vi "test_fpga_scanEngineCore.vi"() -> ()   [LabVIEW 2016]
uses:
  <vilib>/Platform/TimedLoop/XDataNode/wakeup.ctl
  <vilib>/Platform/TimedLoop/XDataNode/XDNodeRunTimeDep.lvlib
  <vilib>/Platform/TimedLoop/XDataNode/nitl_modes.ctl
  <vilib>/Platform/TimedLoop/XDataNode/timing_clust.ctl
  <vilib>/Platform/TimedLoop/XDataNode/XDataNode.xnode
  <vilib>/eio/EIONode/EIONode.xnode
  <vilib>/rvi/FXPMathLib/FxpInterpret/XNode/nifxpmath_Interpret.xnode
  <instrlib>/_niInstr/Basic Elements/v1/FPGA/niInstr Basic Elements v1 FPGA.lvlib
  <vilib>/rvi/FXPMathLib/FxpSub/XNode/nifxpmath_Sub.xnode
  <vilib>/rvi/FXPMathLib/sim/FxpSim.dll
  <vilib>/rvi/FXPMathLib/FxpMul/XNode/nifxpmath_Multiplier.xnode
  <vilib>/rvi/FXPMathLib/FxpAdd/XNode/nifxpmath_Add.xnode
  <vilib>/rvi/DataTransferAndStorage/Container/XNode/niFpgaContainer.xnode
  <vilib>/rvi/FIFO/Fifo_Resource/nirvififoEmulationWrite.vi
  <vilib>/rvi/eio/common/nirviEmuTemplateMethod_errors.vi
  <vilib>/rvi/DataTransferAndStorage/Register/Emulation/niFpgaRegisterEmulation.vi
panel:
  out "pixelEvent":bool
  out "fastIndices":cluster{"index":u16, "next":u16}
  out "indices":T1
  out "outputValid":cluster{"scanValid":bool, "slowValid":bool}
  in  "doSlowMoveFIFO":bool
  out "output":T2
  out "clocks":T3
  out "savedPoint":T4
  out "slowIndices":cluster{"index":u16, "f":u16}
  in  "scanEnabled":bool
  in  "fastDecFactorInv":fxp<+,16,0>
  in  "slowUpStep":fxp<+,22,0>
  in  "outWaveSizeSlow":u16
  in  "scanOffset":cluster{"x":fxp<+/-,16,1>, "y":fxp<+/-,16,1>}
  in  "singleDirectionScan":bool
  in  "moveToPoint":cluster{"x":fxp<+/-,16,1>, "y":fxp<+/-,16,1>}
  in  "invMoveToDec":fxp<+,16,0>
  out "slowMoving":bool
  in  "outputMatrix":T5
  in  "frioRecordingEnable":bool=TRUE
  in  "scanSize":T6
  in  "scanRates":T7={"outputRate"=50, "fastDecFactor"=0, "outWaveSizeFast"=0, "pplUpsampling"=0, "numLines"=0}
  in  "moveRates":T8
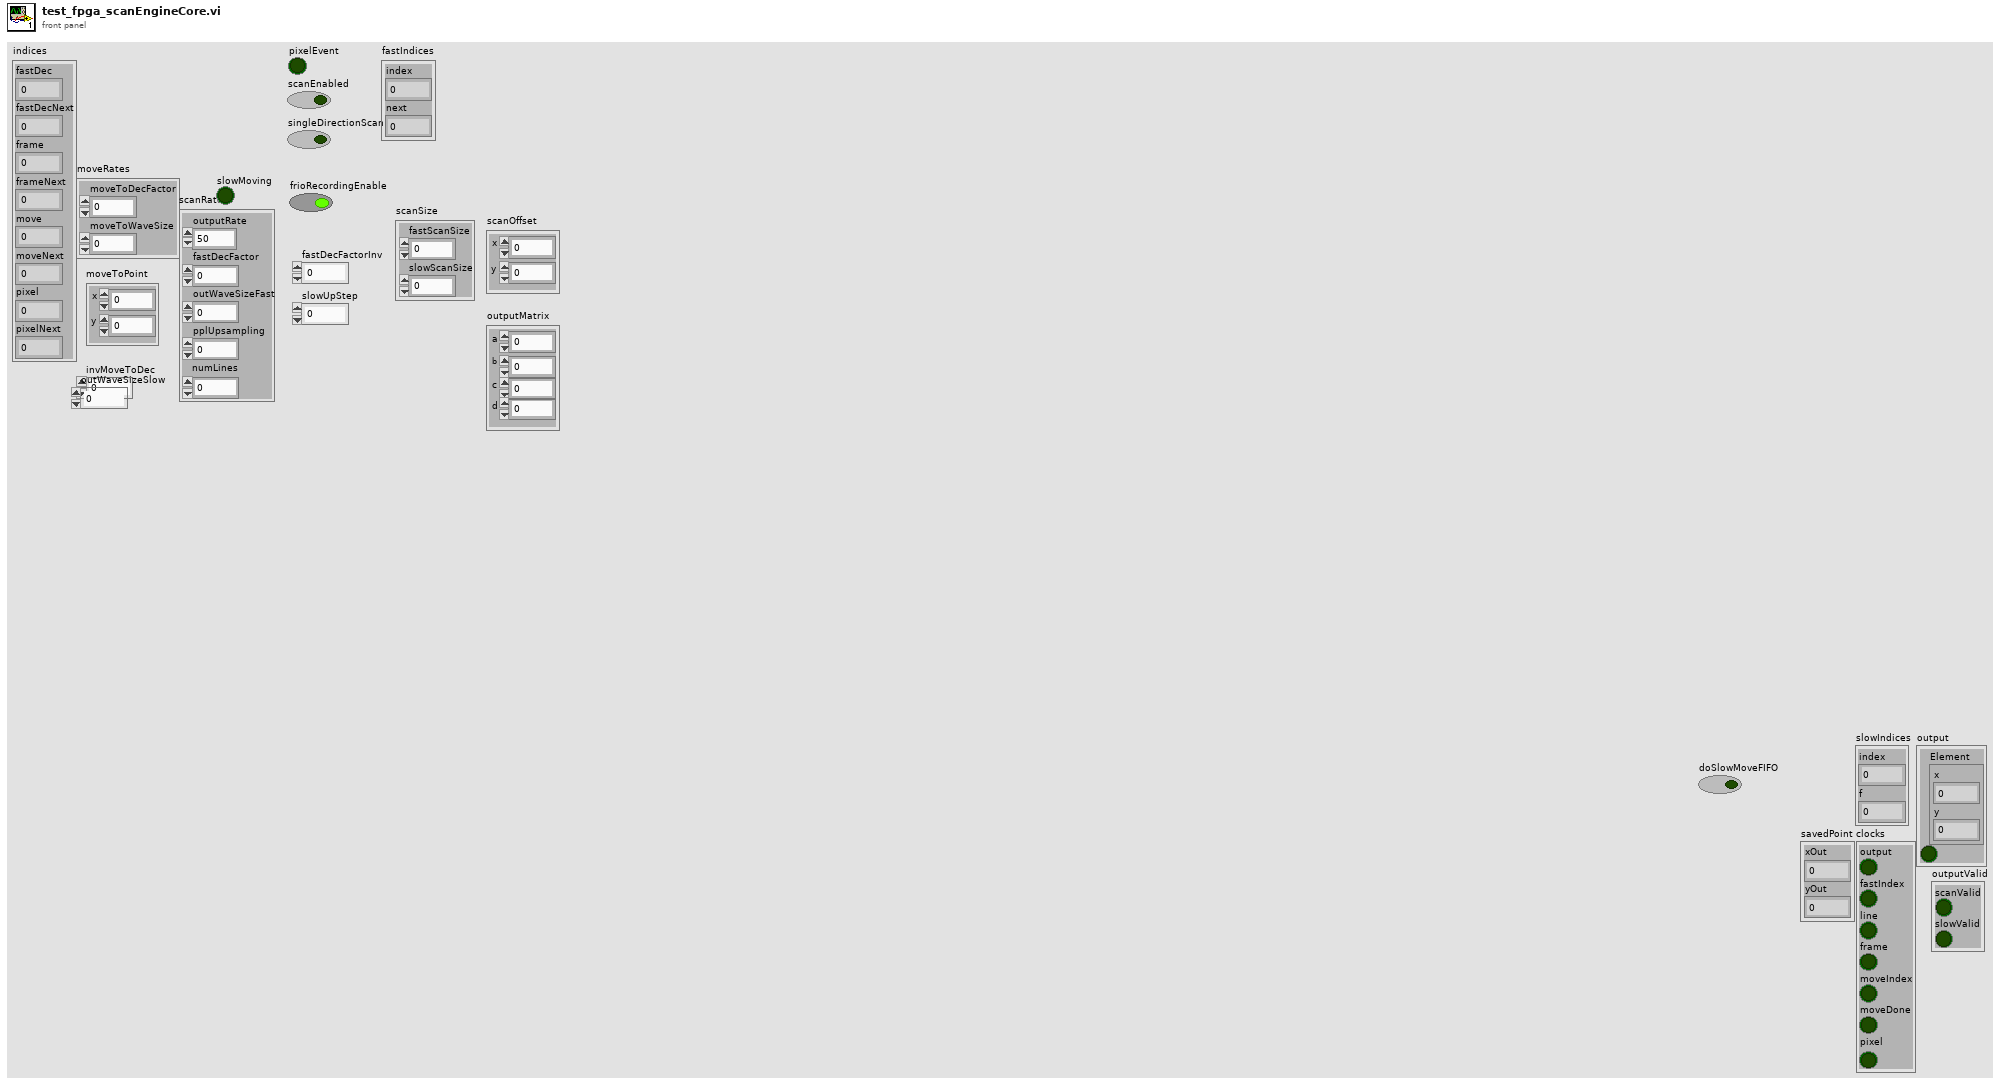
[diagram p1: front panel]
types:
  T1 = cluster{"fastDec":u16, "fastDecNext":u16, "frame":u16, "frameNext":u16, "move":u16, "moveNext":u16, "pixel":u16, "pixelNext":u16}
  T2 = cluster{"Element":cluster{"x":i16, "y":i16}, bool}
  T3 = cluster{"output":bool, "fastIndex":bool, "line":bool, "frame":bool, "moveIndex":bool, "moveDone":bool, "pixel":bool}
  T4 = cluster{"xOut":fxp<+/-,18,2>, "yOut":fxp<+/-,18,2>}
  T5 = cluster{"a":fxp<+/-,18,2>, "b":fxp<+/-,18,2>, "c":fxp<+/-,18,2>, "d":fxp<+/-,18,2>}
  T6 = cluster{"fastScanSize":fxp<+,17,1>, "slowScanSize":fxp<+,17,1>}
  T7 = cluster{"outputRate":u16, "fastDecFactor":u16, "outWaveSizeFast":u16, "pplUpsampling":u16, "numLines":u16}
  T8 = cluster{"moveToDecFactor":u16, "moveToWaveSize":u16}
  T9 = typedef "XDNodeRunTimeDep.lvlib/timing_clust.ctl" = cluster{"Expected End [f-1]":u64, "Actual End [f-1]":u64, "Finished Late? [f-1]":bool, "Expected End [i-1]":u64, "Actual End [i-1]":u64, "Finished Late? [i-1]":bool, "Expected Start [i]":u64, "Actual Start [i]":u64, "Expected Start [f]":u64, "Actual Start [f]":u64, "Source Name":string, "Structure Name":string, "Period":i64, "Deadline":i64, "Offset":i64, "Start":i64, "Priority":i32, "Timeout":i32, "Mode":T10, "Wakeup Reason":T11, "Error":errorcluster, "Source Type":string, "Secondary Source Type":string, "Global End Time":u64, "Global Start Time":u64, "Frame Duration":u64, "Iteration Duration":u64, "Assigned CPU":i32, "I/O Scan Engine Mode":u32}
  T10 = typedef "XDNodeRunTimeDep.lvlib/nitl_modes.ctl" = enum32{"No Change", "Process missed periods, maintain original phase", "Discard missed periods, maintain original phase", "Process missed periods, ignore original phase", "Discard missed periods, ignore original phase"}
  T11 = typedef "XDNodeRunTimeDep.lvlib/wakeup.ctl" = enum32{"Normal", "Aborted", "Asynchronous wakeup", "Timing source error", "Timed loop error", "Timeout"}
  T12 = cluster{"fastDec":u16, "fastDecNext":u16, "frame":u16, "frameNext":u16, "move":u16, "moveNext":u16, "pixel":u16, "pixelNext":u16, "blanking":u32, "blankingNext":u32}
  T13 = cluster{"index":u16, "next":u16, "blanking":u32, "blankingNext":u32}
  T14 = cluster{"x-y":fxp<+/-,18,2>, "x-y":fxp<+/-,18,2>}
  T15 = cluster{"interpOutput":fxp<+/-,19,2>, "interpOutput":fxp<+/-,19,2>}
  T16 = cluster{"x+y":fxp<+/-,18,2>, "x+y":fxp<+/-,18,2>}
  T17 = cluster{"edge detected":bool, "output valid":bool}
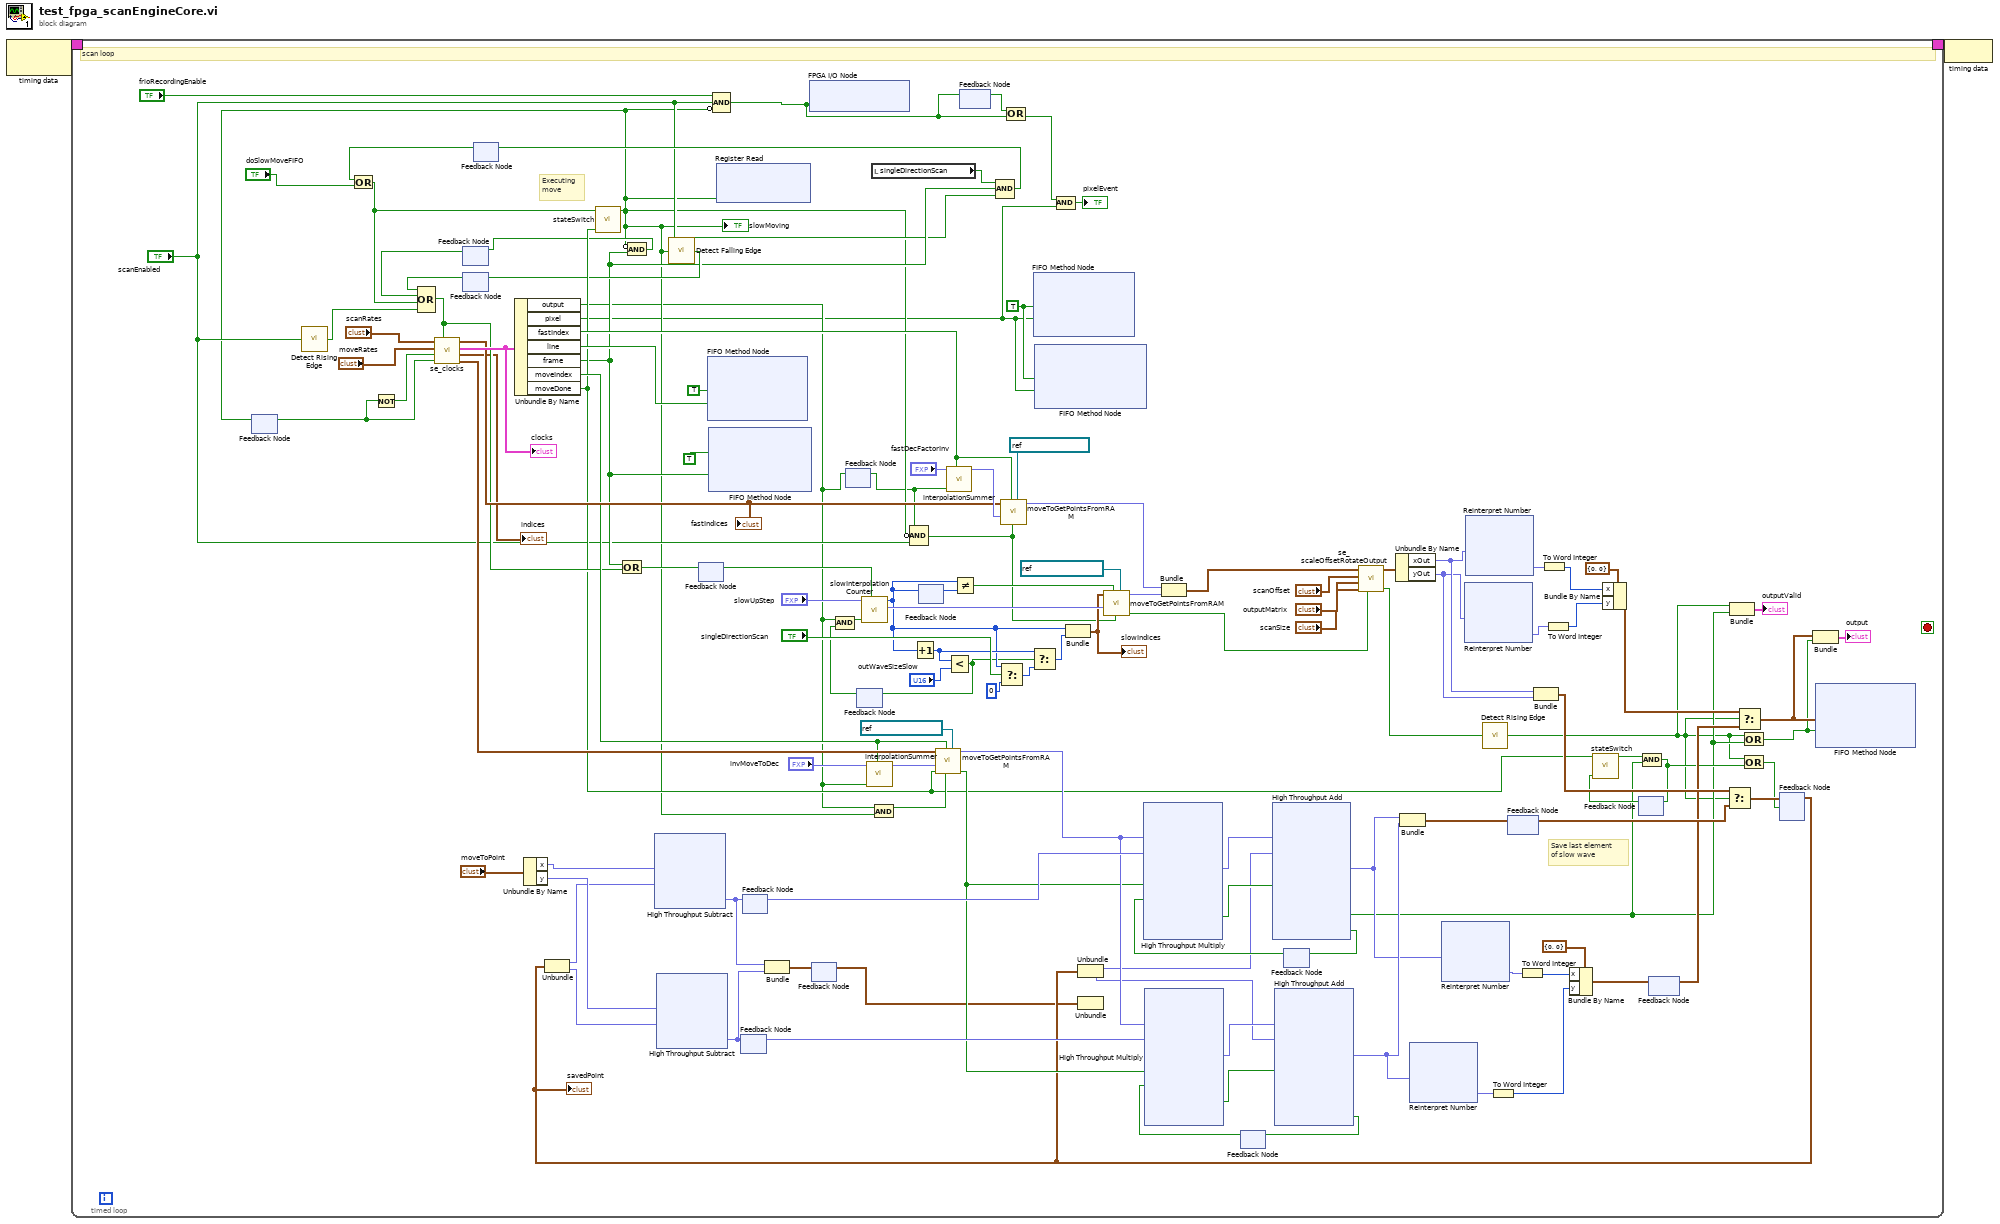
[diagram p0: block diagram]
diagram:
  n1 = node-c288() -> (w2:T9)  [unwired: 1 in]
  n2 = timed-loop {
    timing: w2 -> [_]
    timing-out: [_] -> w1
    stop <- _ stop-if-true
    w82 = TRUE ("Element")
    # "Save last element \nof slow wave"
    # "Executing\nmove"
    # "scan loop"
    n3 = feedback #1() -> (w17:bool)  [unwired: 1 in]
    n4 = call <instrlib>:"Detect Rising Edge.vi"("signal"="scanEnabled") -> ("edge detected"=w65:bool)  [unwired: 14 in]
    n5 = Not(x=w17) -> (.not. x?=w16:bool)
    n6 = feedback #2() -> (w64:bool)  [unwired: 1 in]
    n7 = feedback #3() -> (w63:bool)  [unwired: 1 in]
    n8 = feedback #4() -> (w33:bool)  [unwired: 1 in]
    n9 = Compound Arithmetic op=OR(w33, "doSlowMoveFIFO") -> (w28:bool)
    n10 = Compound Arithmetic op=OR(w63, w64, w28, w65) -> (w31:bool)
    n11 = call "se_clocks.vi"("se.p.resetClocks"=w31, "stepSlow"=w17, "stepScan"=w16, "moveRates"="moveRates", "se.p.clocks"="scanRates") -> ("moveIndices"=w73:cluster{"index":u16, "next":u16}, "indices"=→"indices":T12, "clocks"=w77:T3, "fastIndices"=w75:T13)  [unwired: 3 in]
    "clocks" <- w77
    "fastIndices" <- w75
    n12 = Unbundle By Name(w77) -> ("output"=w9:bool, "pixel"=w7:bool, "fastIndex"=w72:bool, "line"=w76:bool, "frame"=w27:bool, "moveIndex"=w71:bool, "moveDone"=w30:bool)
    n13 = Unbundle By Name("moveToPoint") -> ("x"=w103:fxp<+/-,16,1>, "y"=w104:fxp<+/-,16,1>)
    n14 = call "stateSwitch.vi"("disable"=w30, "enable"=w28) -> ("state"=w14:bool)  [unwired: 9 in]
    "slowMoving" <- w14
    n15 = feedback-in #1(w14) -> ()
    n16 = Compound Arithmetic op=OR(w27, w31) -> (w32:bool)
    n17 = Compound Arithmetic op=AND(invert w14, w27) -> (w26:bool)
    n18 = feedback-in #2(w26) -> ()
    n19 = call <instrlib>:"Detect Falling Edge.vi"("signal"=w14) -> ("edge detected"=w29:bool)  [unwired: 14 in]
    n20 = feedback-in #3(w29) -> ()
    n21 = feedback-in #5(w32) -> ()
    n22 = feedback #5() -> (w10:bool)  [unwired: 1 in]
    n23 = xnode ("FIFO Method Node")("Element"=TRUE, "Input Valid"=w76) -> ()  [unwired: 1 in, 2 out]
    n24 = xnode ("FIFO Method Node")("Element"=TRUE, "Input Valid"=w27) -> ()  [unwired: 1 in, 2 out]
    n25 = Compound Arithmetic op=AND("frioRecordingEnable", "scanEnabled", invert w14) -> (w4:bool)
    n26 = xnode ("Register Read")("Data"=w14) -> ()  [unwired: 1 in, 1 out]
    n27 = feedback #6() -> (w114:fxp<+/-,18,2>)  [unwired: 1 in]
    n28 = feedback #7() -> (w111:fxp<+/-,18,2>)  [unwired: 1 in]
    n29 = xnode "FPGA I/O Node"("outputEnabled"=w4) -> ()  [unwired: 1 in, 1 out]
    n30 = feedback #8() -> (w43:T14)  [unwired: 1 in]
    n31 = feedback #9() -> (w8:bool)  [unwired: 1 in]
    n32 = feedback-in #9(w9) -> ()
    n33 = feedback #10() -> (w11:bool)  [unwired: 1 in]
    n34 = Compound Arithmetic op=AND(w9, w11) -> (w13:bool)
    n35 = call "slowInterpolationCounter.vi"("reset"=w10, "doStep"=w13, "upStep"="slowUpStep") -> ("fraction"=w80:fxp<+,28,0>, "index"=w67:u16)  [unwired: 7 in]
    n36 = call "interpolationSummer.vi"("reset"=w71, "doStep"=w9, "upStep"="invMoveToDec") -> ("position"=w98:fxp<+,22,0>)  [unwired: 8 in]
    n37 = local read "singleDirectionScan"() -> (w35:bool)
    n38 = Compound Arithmetic op=AND(w9, w14) -> (w42:bool)
    n39 = Compound Arithmetic op=AND(w8, invert w14, "scanEnabled") -> (w41:bool)
    n40 = Increment(x=w67) -> (x+1=w95:u16)
    n41 = feedback-in #11(w67) -> ()
    n42 = feedback #11() -> (w68:u16)  [unwired: 1 in]
    n43 = call "moveToGetPointsFromRAM.vi"("Memory In"=refnum<k21> "moveToWave", "inputValid"=w42, "reset"=w71, "maxReached"=w30, "interpPosition"=w98, "adresses"=w73) -> ("outputValid"=w51:bool, "interpOutput"=w97:fxp<+/-,19,2>)  [unwired: 4 in]
    n44 = call "interpolationSummer.vi"("reset"=w72, "doStep"=w8, "upStep"="fastDecFactorInv") -> ("position"=w87:fxp<+,22,0>)  [unwired: 8 in]
    n45 = Less?(x=w95, y="outWaveSizeSlow") -> (x < y?=w12:bool)
    n46 = feedback-in #10(w12) -> ()
    n47 = Not Equal?(x=w67, y=w68) -> (x != y?=w66:bool)
    n48 = feedback-in #12(w4) -> ()
    n49 = feedback #12() -> (w3:bool)  [unwired: 1 in]
    n50 = Compound Arithmetic op=AND(w35, w27, "scanEnabled") -> (w34:bool)
    n51 = feedback-in #4(w34) -> ()
    n52 = Select(t=w67, s="singleDirectionScan", f=u16 0) -> (s? t:f=w94:u16)
    n53 = call "moveToGetPointsFromRAM.vi"("Memory In"=refnum<k21> "fastAxisWave", "inputValid"=w41, "reset"=w72, "interpPosition"=w87, "adresses"=w75) -> ("interpOutput"=w85:fxp<+/-,19,2>)  [unwired: 5 in, 1 out]
    n54 = Compound Arithmetic op=OR(w3, w4) -> (w5:bool)
    n55 = Select(t=w95, s=w12, f=w94) -> (s? t:f=w81:u16)
    n56 = xnode ("FIFO Method Node")("Element"=w82, "Input Valid"=w7) -> ()  [unwired: 1 in, 2 out]
    n57 = xnode ("FIFO Method Node")("Element"=w82, "Input Valid"=w7) -> ()  [unwired: 1 in, 2 out]
    n58 = Compound Arithmetic op=AND(w5, w7) -> (→"pixelEvent":bool)
    n59 = Bundle("index"=w67, "f"=w81) -> (w69:cluster{"index":u16, "f":u16})  [unwired: 1 in]
    "slowIndices" <- w69
    n60 = Unbundle(w43) -> ()  [unwired: 2 out]
    n61 = call "moveToGetPointsFromRAM.vi"("Memory In"=refnum<k21> "slowAxisWave", "inputValid"=w41, "reset"=w66, "interpPosition"=w80, "adresses"=w69) -> ("outputValid"=w70:bool, "interpOutput"=w84:fxp<+/-,19,2>)  [unwired: 5 in]
    n62 = Bundle("interpOutput"=w85, "interpOutput"=w84) -> (w83:T15)  [unwired: 1 in]
    n63 = feedback #13() -> (w107:bool)  [unwired: 1 in]
    n64 = xnode ("High Throughput Multiply")("x"=w97, "y"=w114, "input valid"=w51, "ready for output (T)"=w107) -> ("x*y"=w113:fxp<+/-,18,2>, "output valid"=w115:bool)  [unwired: 1 out]
    n65 = feedback #14() -> (w109:bool)  [unwired: 1 in]
    n66 = xnode ("High Throughput Multiply")("x"=w97, "y"=w111, "input valid"=w51, "ready for output (T)"=w109) -> ("x*y"=w112:fxp<+/-,18,2>, "output valid"=w110:bool)  [unwired: 1 out]
    n67 = call "se_scaleOffsetRotateOutput.vi"("inputValid"=w70, "scanSize"="scanSize", "outputMatrix"="outputMatrix", "scanOffset"="scanOffset", "input"=w83) -> ("outputValid"=w93:bool, "outputNorm"=w92:T4)  [unwired: 4 in, 1 out]
    n68 = Unbundle By Name(w92) -> ("xOut"=w58:fxp<+/-,18,2>, "yOut"=w57:fxp<+/-,18,2>)
    n69 = xnode "Reinterpret Number"("x"=w57) -> ("y"=w128:fxp<+/-,18,17>)
    n70 = xnode "Reinterpret Number"("x"=w58) -> ("y"=w129:fxp<+/-,18,17>)
    n71 = call <instrlib>:"Detect Rising Edge.vi"("signal"=w93) -> ("edge detected"=w19:bool)  [unwired: 14 in]
    n72 = feedback #15() -> (w50:T16)  [unwired: 1 in]
    n73 = Bundle("xOut"=w58, "yOut"=w57) -> (w56:T4)  [unwired: 1 in]
    n74 = To Word Integer(number=w129) -> (16bit integer=w126:i16)
    n75 = To Word Integer(number=w128) -> (16bit integer=w125:i16)
    n76 = Bundle By Name(cluster=cluster{"x":i16, "y":i16} {"x"=0, "y"=0} ("Element"), "x"=w126, "y"=w125) -> (w62:cluster{"x":i16, "y":i16})
    n77 = feedback #16() -> (w38:bool)  [unwired: 1 in]
    n78 = call "stateSwitch.vi"("disable"=w38, "enable"=w30) -> ("state"=w39:bool)  [unwired: 9 in]
    n79 = feedback #17() -> (w40:cluster{"x":i16, "y":i16})  [unwired: 1 in]
    n80 = Select(t=w56, s=w19, f=w50) -> (s? t:f=w54:T16)
    n81 = Select(t=w62, s=w19, f=w40) -> (s? t:f=w24:cluster{"x":i16, "y":i16})
    n82 = feedback #18() -> (w49:T4)  [unwired: 1 in]
    "savedPoint" <- w49
    n83 = Unbundle(w49) -> ("xOut"=w52:fxp<+/-,18,2>, "yOut"=w53:fxp<+/-,18,2>)
    n84 = xnode "High Throughput Subtract"("x"=w103, "y"=w52) -> ("x-y"=w46:fxp<+/-,18,2>)
    n85 = xnode "High Throughput Subtract"("x"=w104, "y"=w53) -> ("x-y"=w45:fxp<+/-,18,2>)
    n86 = feedback-in #6(w45) -> ()
    n87 = feedback-in #7(w46) -> ()
    n88 = Bundle("x-y"=w46, "x-y"=w45) -> (w44:T14)  [unwired: 1 in]
    n89 = feedback-in #8(w44) -> ()
    n90 = Unbundle(w49) -> ("xOut"=w47:fxp<+/-,18,2>, "yOut"=w48:fxp<+/-,18,2>)
    n91 = xnode ("High Throughput Add")("x"=w112, "y"=w47, "input valid"=w110) -> ("x+y"=w59:fxp<+/-,18,2>, "output valid"=w20:bool, "ready for input"=w108:bool)  [unwired: 1 in]
    n92 = xnode ("High Throughput Add")("x"=w113, "y"=w48, "input valid"=w115) -> ("x+y"=w60:fxp<+/-,18,2>, "ready for input"=w106:bool)  [unwired: 1 in, 1 out]
    n93 = feedback-in #13(w106) -> ()
    n94 = feedback-in #14(w108) -> ()
    n95 = Bundle("x+y"=w59, "x+y"=w60) -> (w55:T16)  [unwired: 1 in]
    n96 = xnode "Reinterpret Number"("x"=w60) -> ("y"=w116:fxp<+/-,18,17>)
    n97 = xnode "Reinterpret Number"("x"=w59) -> ("y"=w119:fxp<+/-,18,17>)
    n98 = To Word Integer(number=w116) -> (16bit integer=w118:i16)
    n99 = feedback-in #15(w55) -> ()
    n100 = To Word Integer(number=w119) -> (16bit integer=w120:i16)
    n101 = Bundle By Name(cluster=cluster{"x":i16, "y":i16} {"x"=0, "y"=0} ("Element"), "x"=w120, "y"=w118) -> (w61:cluster{"x":i16, "y":i16})
    n102 = Compound Arithmetic op=AND(w39, w20) -> (w37:bool)
    n103 = feedback-in #16(w37) -> ()
    n104 = feedback-in #17(w61) -> ()
    n105 = Bundle("edge detected"=w19, "output valid"=w20) -> (→"outputValid":T17)  [unwired: 1 in]
    n106 = Compound Arithmetic op=OR(w19, w20) -> (w23:bool)
    n107 = Compound Arithmetic op=OR(w19, w37) -> (w36:bool)
    n108 = feedback-in #18(w54, w36) -> ()
    n109 = Bundle("Element"=w24, w23) -> (→"output":T2)  [unwired: 1 in]
    n110 = xnode ("FIFO Method Node")("Element"=w24, "Input Valid"=w23) -> ()  [unwired: 1 in, 2 out]
  }
  n111 = node-c288(w1) -> ()
